vi "Untitled 7.vi"() -> ()   [LabVIEW 2017]
uses:
  Global 1.vi
panel:
  in  "stop 2":bool
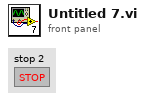
[diagram p1: front panel]
types:
  T1 = enum16{"Standard", "Buffered", "CRLF", "Immediate"}
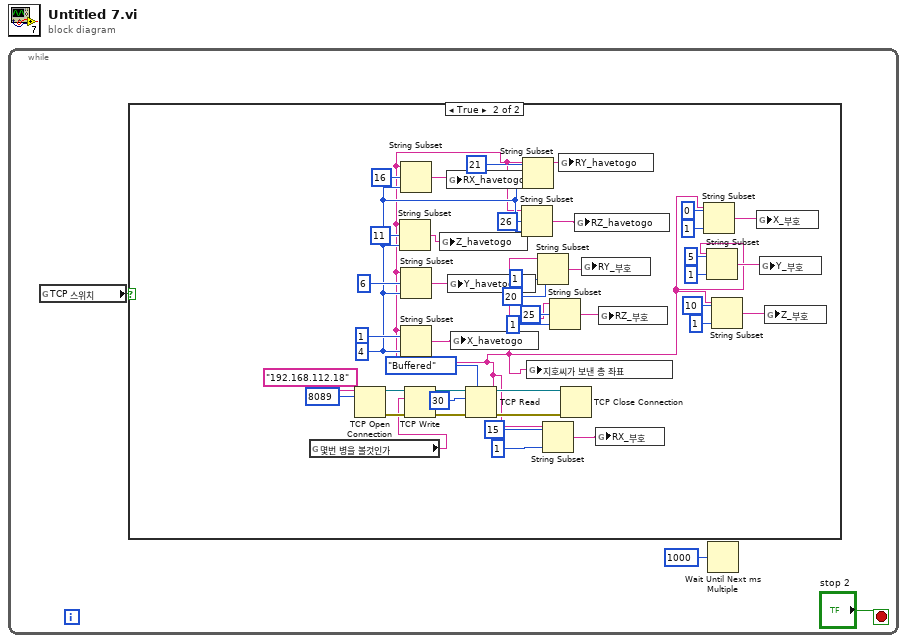
[diagram p0: block diagram]
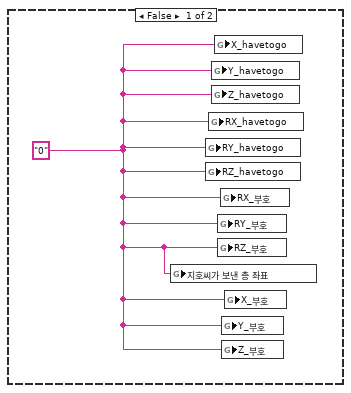
[diagram p2: hidden frame]
diagram:
  n1 = while {
    stop <- "stop 2" stop-if-true
    n2 = global read "Global 1.vi" "TCP 스위치"() -> (w2:bool)
    n3 = case shown="True" w2 {
      frame False {
        w4 = "0"
        n4 = global write "Global 1.vi" "지호씨가 보낸 총 좌표"(w4) -> ()
        n5 = global write "Global 1.vi" "RY_havetogo"(w4) -> ()
        n6 = global write "Global 1.vi" "RZ_havetogo"(w4) -> ()
        n7 = global write "Global 1.vi" "RX_havetogo"(w4) -> ()
        n8 = global write "Global 1.vi" "Y_havetogo"(w4) -> ()
        n9 = global write "Global 1.vi" "Z_havetogo"(w4) -> ()
        n10 = global write "Global 1.vi" "X_havetogo"(w4) -> ()
        n11 = global write "Global 1.vi" "RY_부호"(w4) -> ()
        n12 = global write "Global 1.vi" "RZ_부호"(w4) -> ()
        n13 = global write "Global 1.vi" "RX_부호"(w4) -> ()
        n14 = global write "Global 1.vi" "Y_부호"(w4) -> ()
        n15 = global write "Global 1.vi" "Z_부호"(w4) -> ()
        n16 = global write "Global 1.vi" "X_부호"(w4) -> ()
      }
      frame True {
        w41 = 4 ("length (rest)")
        n17 = global read "Global 1.vi" "몇번 병을 볼것인가"() -> (w32:string)
        n18 = TCP Open Connection(address="192.168.112.18", remote port or service name=u16 8089) -> (connection ID=w36:refnum<k5>, error out=w35:errorcluster)  [unwired: 3 in]
        n19 = TCP Write(connection ID=w36, data in=w32, error in (no error)=w35) -> (connection ID out=w34:refnum<k5>, error out=w33:errorcluster)  [unwired: 1 in, 1 out]
        n20 = TCP Read(connection ID=w34, bytes to read=30, error in (no error)=w33, 7:T1."Buffered" ("mode (standard)")) -> (connection ID out=w45:refnum<k5>, data out=w5:string, error out=w44:errorcluster)  [unwired: 1 in]
        n21 = String Subset(string=w5, offset (0)=11, length (rest)=w41) -> (substring=w23:string)
        n22 = String Subset(string=w5, offset (0)=16, length (rest)=w41) -> (substring=w22:string)
        n23 = String Subset(string=w5, offset (0)=6, length (rest)=w41) -> (substring=w24:string)
        n24 = String Subset(string=w5, offset (0)=1, length (rest)=w41) -> (substring=w25:string)
        n25 = global write "Global 1.vi" "Z_havetogo"(w23) -> ()
        n26 = global write "Global 1.vi" "RX_havetogo"(w22) -> ()
        n27 = global write "Global 1.vi" "Y_havetogo"(w24) -> ()
        n28 = global write "Global 1.vi" "X_havetogo"(w25) -> ()
        n29 = String Subset(string=w5, offset (0)=26, length (rest)=w41) -> (substring=w20:string)
        n30 = String Subset(string=w5, offset (0)=21, length (rest)=w41) -> (substring=w21:string)
        n31 = global write "Global 1.vi" "지호씨가 보낸 총 좌표"(w5) -> ()
        n32 = String Subset(string=w5, offset (0)=20, length (rest)=1 ("length (rest)")) -> (substring=w18:string)
        n33 = String Subset(string=w5, offset (0)=15, length (rest)=1 ("length (rest)")) -> (substring=w19:string)
        n34 = String Subset(string=w5, offset (0)=25, length (rest)=1 ("length (rest)")) -> (substring=w17:string)
        n35 = global write "Global 1.vi" "RY_havetogo"(w21) -> ()
        n36 = TCP Close Connection(connection ID=w45, error in (no error)=w44) -> ()  [unwired: 1 in, 2 out]
        n37 = global write "Global 1.vi" "RZ_havetogo"(w20) -> ()
        n38 = global write "Global 1.vi" "RY_부호"(w18) -> ()
        n39 = global write "Global 1.vi" "RX_부호"(w19) -> ()
        n40 = global write "Global 1.vi" "RZ_부호"(w17) -> ()
        n41 = String Subset(string=w5, offset (0)=0, length (rest)=1 ("length (rest)")) -> (substring=w14:string)
        n42 = String Subset(string=w5, offset (0)=5, length (rest)=1 ("length (rest)")) -> (substring=w11:string)
        n43 = String Subset(string=w5, offset (0)=10, length (rest)=1 ("length (rest)")) -> (substring=w8:string)
        n44 = global write "Global 1.vi" "X_부호"(w14) -> ()
        n45 = global write "Global 1.vi" "Y_부호"(w11) -> ()
        n46 = global write "Global 1.vi" "Z_부호"(w8) -> ()
      }
    }
    n47 = Wait Until Next ms Multiple(millisecond multiple=u32 1000) -> ()  [unwired: 1 out]
  }
